vi "2013_02_13 Durability8 Main.vi"() -> ()   [LabVIEW 2012]
uses:
  MotorTypeDef.ctl
  <vilib>/DAQmx/write.llb/DAQmx Write (Counter Time 1Chan 1Samp).vi
  <vilib>/DAQmx/read.llb/DAQmx Read (Analog 1D Wfm NChan NSamp).vi
  <vilib>/Utility/TradDaqScaling.llb/Convert Thermistor Reading (waveform).vi
  <vilib>/DAQmx/miscellaneous.llb/DAQmx Fill In Error Info.vi
  <resource>/objmgr/daqmx.rc
panel:
  out "TotalSampPerChanAcquired":dbl
  out "AvailSampPerChan":u32
  in  "Y axis":u16(ring)=3 items=["RMS Current (A) 1"=1, "RMS Voltage (V) 1"=2, "RPM"=3, "Supply (V)"=4, "Torque (mNm)"=5, "Electrical Power (W)"=6, "Mechanical Power(W)"=7, "Motor Efficiency (%)"=8, "Source Current (A)"=10, "Supply Power (W)"=11, "ESC Efficiency (%)"=12, "Flow"=13, "Pressure Blue"=14, "Pressure Yellow"=15, "etc"=16]
  in  "X axis":u16(ring) items=["RMS Current (A) 1"=1, "RMS Voltage (V) 1"=2, "RPM"=3, "Supply (V)"=4, "Torque (mNm)"=5, "Electrical Power (W)"=6, "Mechanical Power(W)"=7, "Motor Efficiency (%)"=8, "Source Current (A)"=10, "Supply Power (W)"=11, "ESC Efficiency (%)"=12, "Flow"=13, "Pressure Blue"=14, "Pressure Yellow"=15, "Elapsed Time (s)"=0]
  out "XY Graph 2":cluster{"Array":dbl[], "Array":dbl[]}[](graph)
  out "Single Motor 2":waveform(dbl)[](graph)
  in  "Waveform":bool
  in  "Motor":dbl=1.0 min=1.0 max=8.0 step=1.0
  out "XY Graph":cluster{"Array":dbl[], "Array":dbl[]}[](graph)
  out "error out":errorcluster
  in  "File Path":path=path "Durability/.lvm"
  in  "Motor 8":T1 {"Elec Power In (W)" format="%.3g"; "Efficiency" format="%#_3g%%"; "Mech Pwr Out (W)" format="%.3g"; "Torque (mNm)" format="%.3g"; "Elapsed Time" format="%<%H:%M:%S>t"; "Supply (V)" format="%.2f"; "RPM" scale=0.0..40000.0 scale format="%#_4p"}
  in  "Motor 7":T1 {"Elec Power In (W)" format="%.3g"; "Efficiency" format="%#_3g%%"; "Mech Pwr Out (W)" format="%.3g"; "Torque (mNm)" format="%.3g"; "Elapsed Time" format="%<%H:%M:%S>t"; "Supply (V)" format="%.2f"; "RPM" scale=0.0..40000.0 scale format="%#_4p"}
  in  "Motor 6":T1 {"Elec Power In (W)" format="%.3g"; "Efficiency" format="%#_3g%%"; "Mech Pwr Out (W)" format="%.3g"; "Torque (mNm)" format="%.3g"; "Elapsed Time" format="%<%H:%M:%S>t"; "Supply (V)" format="%.2f"; "RPM" scale=0.0..40000.0 scale format="%#_4p"}
  in  "Motor 5":T1 {"Elec Power In (W)" format="%.3g"; "Efficiency" format="%#_3g%%"; "Mech Pwr Out (W)" format="%.3g"; "Torque (mNm)" format="%.3g"; "Elapsed Time" format="%<%H:%M:%S>t"; "Supply (V)" format="%.2f"; "RPM" scale=0.0..40000.0 scale format="%#_4p"}
  in  "Motor 4":T1 {"Elec Power In (W)" format="%.3g"; "Efficiency" format="%#_3g%%"; "Mech Pwr Out (W)" format="%.3g"; "Torque (mNm)" format="%.3g"; "Elapsed Time" format="%<%H:%M:%S>t"; "Supply (V)" format="%.2f"; "RPM" scale=0.0..40000.0 scale format="%#_4p"}
  in  "Motor 3":T1 {"Elec Power In (W)" format="%.3g"; "Efficiency" format="%#_3g%%"; "Mech Pwr Out (W)" format="%.3g"; "Torque (mNm)" format="%.3g"; "Elapsed Time" format="%<%H:%M:%S>t"; "Supply (V)" format="%.2f"; "RPM" scale=0.0..40000.0 scale format="%#_4p"}
  in  "Motor 2":T1 {"Elec Power In (W)" format="%.3g"; "Efficiency" format="%#_3g%%"; "Mech Pwr Out (W)" format="%.3g"; "Torque (mNm)" format="%.3g"; "Elapsed Time" format="%<%H:%M:%S>t"; "Supply (V)" format="%.2f"; "RPM" scale=0.0..40000.0 scale format="%#_4p"}
  in  "Motor 1":T1 {"Elec Power In (W)" format="%.3g"; "Efficiency" format="%#_3g%%"; "Mech Pwr Out (W)" format="%.3g"; "Torque (mNm)" format="%.3g"; "Elapsed Time" format="%<%H:%M:%S>t"; "Supply (V)" format="%.2f"; "RPM" scale=0.0..40000.0 scale format="%#_4p"}
  out "Motor Temp":dbl(slide) scale=65.0..110.0
  out "Tank Temp":dbl(slide) scale=65.0..110.0
  in  "Temp Probe\nOn Motor":dbl=9.0
  out "loop time (ms)":u32
  in  "stop":bool
  in  "Unlock PWM":bool=TRUE
  in  "PWM 2":dbl(slide)=100.0 min=0.0 max=100.0 step=5.0 scale=0.0..100.0
  in  "PWM 1":dbl(slide) min=0.0 max=100.0 step=5.0 scale=0.0..100.0
  # "Enable"
  # "Fail"
  # "Enable"
  # "Fail"
  # "Enable"
  # "Fail"
  # "Enable"
  # "Fail"
  # "Enable"
  # "Fail"
  # "Enable"
  # "Fail"
  # "Enable"
  # "Fail"
  # "Enable"
  # "Fail"
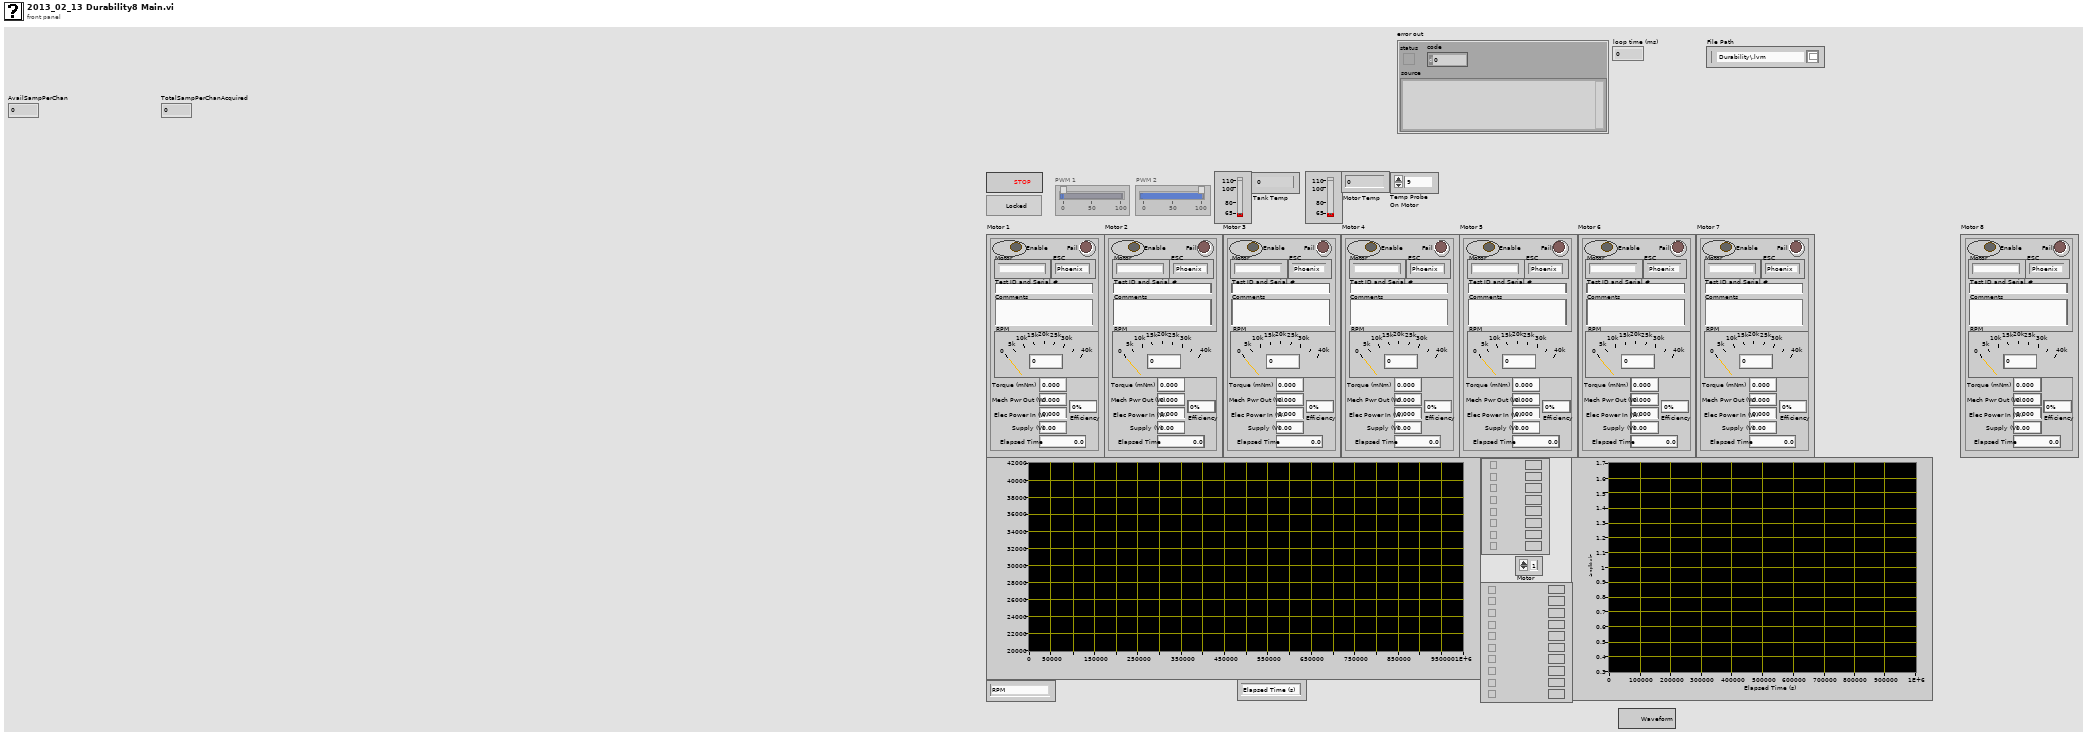
[diagram p1: front panel]
types:
  T1 = typedef "MotorTypeDef.ctl" = cluster{"Enabled":bool, "Fail":bool, "RPM":dbl, "Motor":enum16{"", "Maxon EC6 6V", "Maxon EC4 6V", "FH 0620 6V", "FH 0620 12V"}, "ESC":enum16{"Phoenix", "Maxon", "FH 1801"}, "Supply (V)":dbl, "Test ID and Serial #":string, "Comments":string, "Elapsed Time":dbl, "Counter":dbl, "Torque (mNm)":dbl, "Mech Pwr Out (W)":dbl, "Efficiency":dbl, "Elec Power In (W)":dbl}
  T2 = enum8{"Enabled", "Disabled", "Disabled and Grayed Out"}
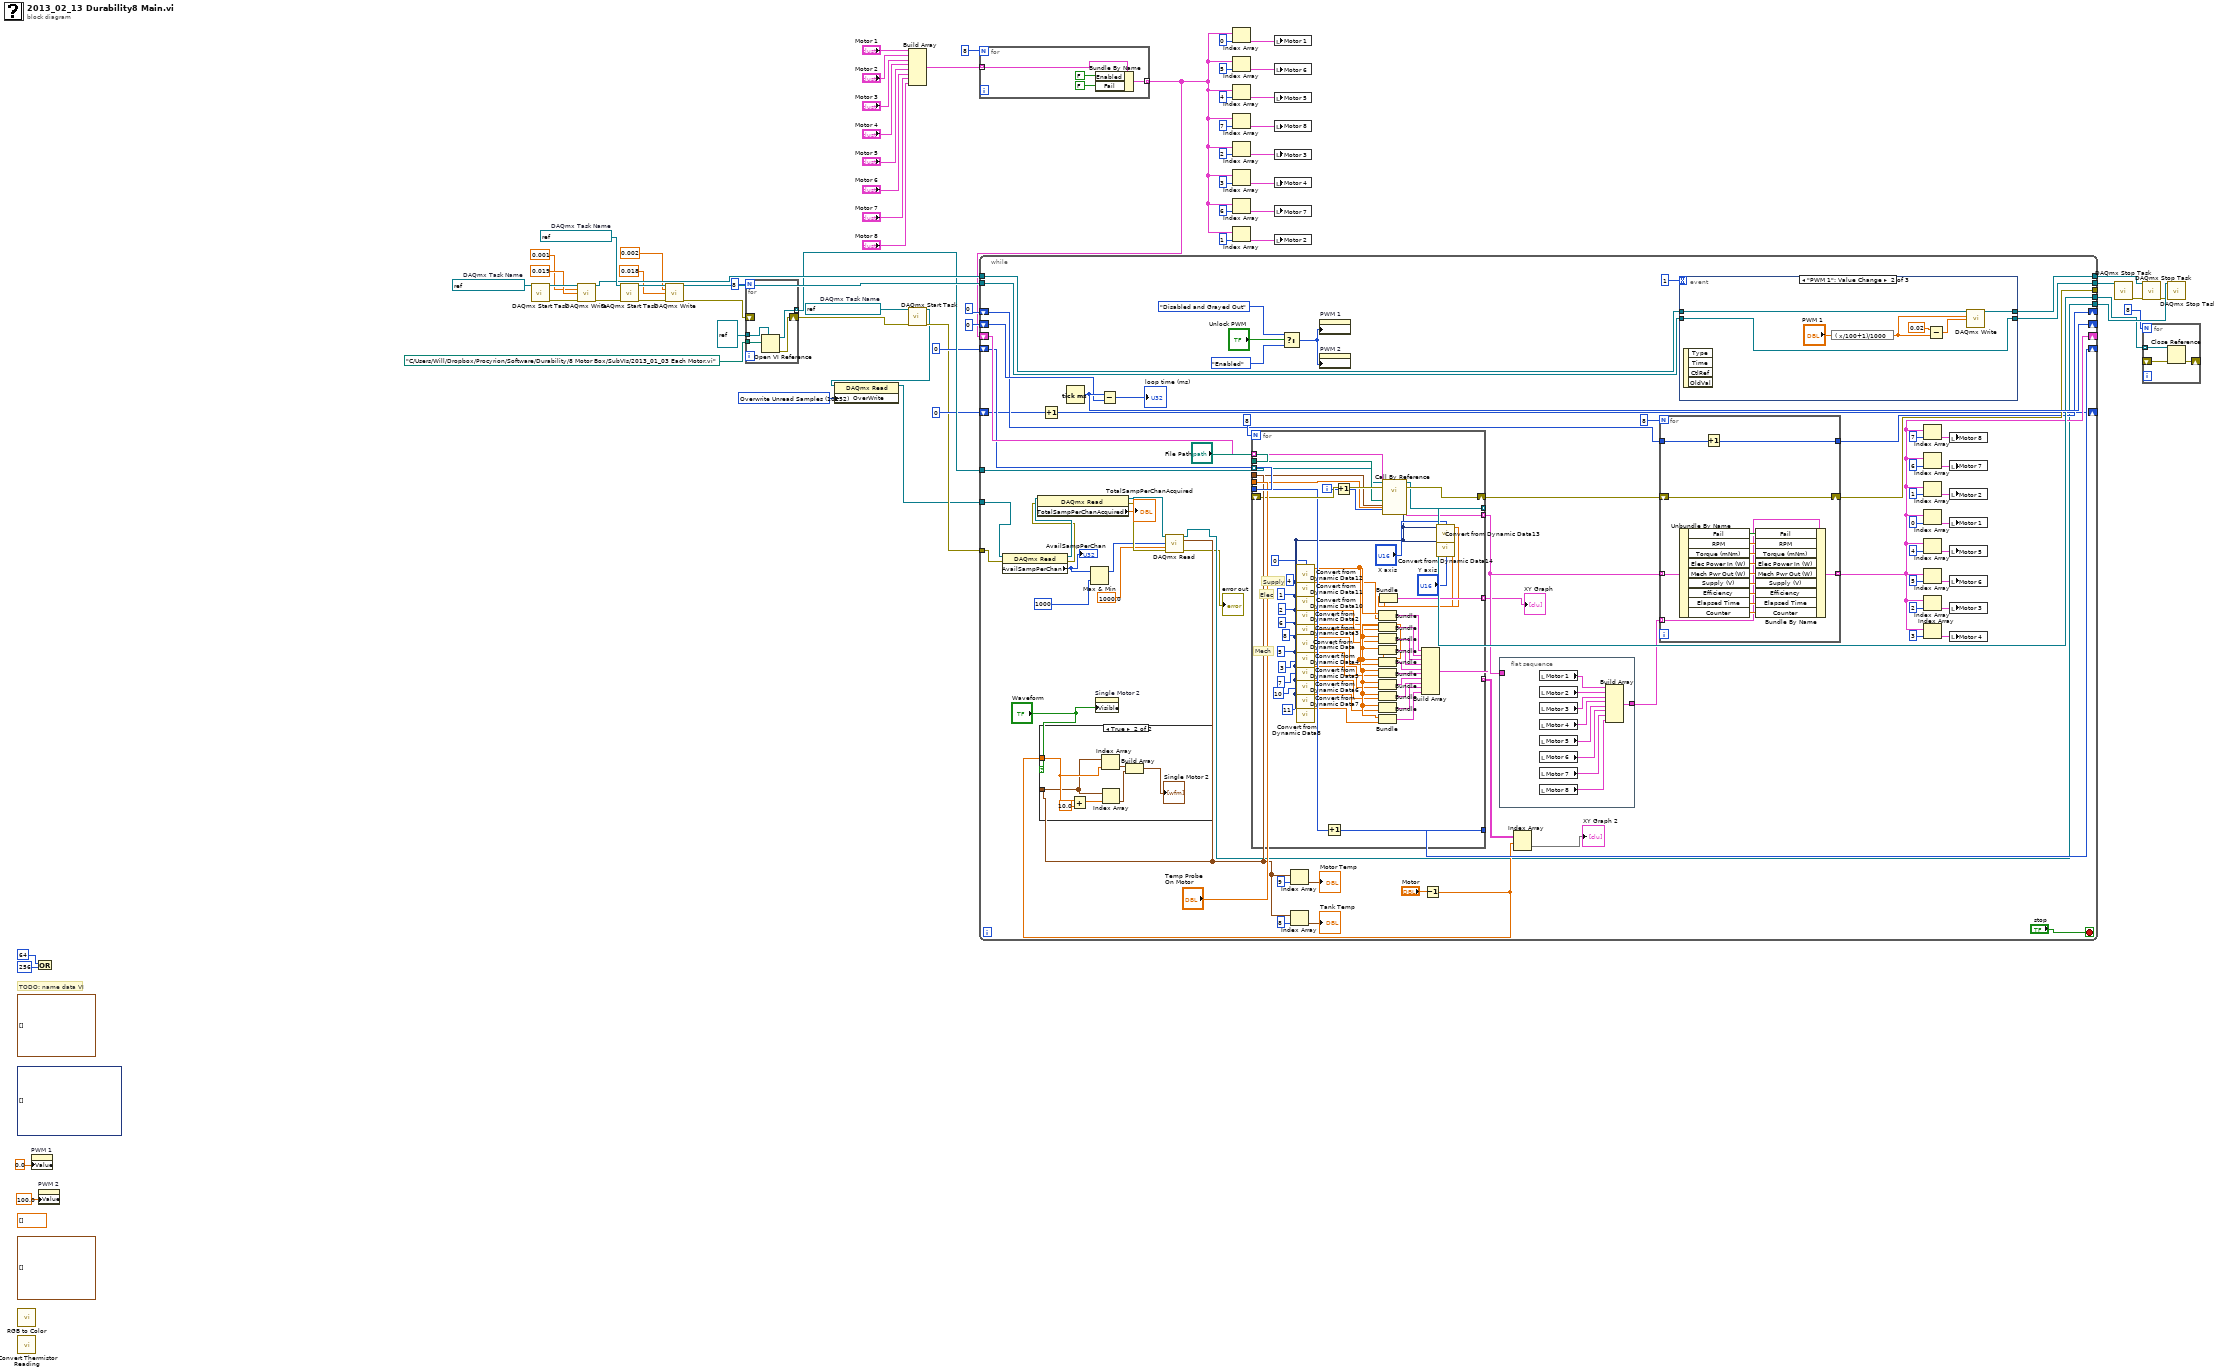
[diagram p0: block diagram]
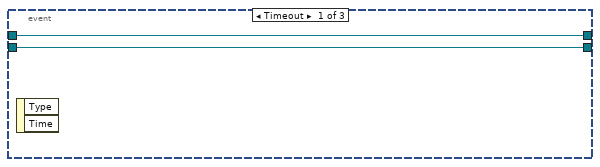
[diagram p3: hidden frame]
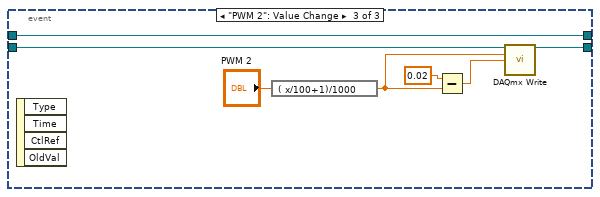
[diagram p4: hidden frame]
diagram:
  w1 = 10252 items=["Overwrite Unread Samples"=10252, "Do Not Overwrite Unread Samples"=10159] ("OverWrite")
  (unwired) dynamicdata[] []
  (unwired) dbl[] [] ("History Data")
  (unwired) waveform(dbl)[][] [] ("History Data")
  (unwired) waveform(dbl)[][] [] ("History Data")
  w63 = refnum<k21> "Durability8 PWM2"  # DAQmx Task Name
  w64 = refnum<k21> "Durability8 PWM1"  # DAQmx Task Name
  w66 = refnum<k21> "Durability8 Acquire"  # DAQmx Task Name
  # "TODO: name data VI"
  n1 = call <vilib>:"RGB to Color.vi"() -> ()  [unwired: 3 in, 1 out]
  n2 = call-poly <vilib>:"Convert Thermistor Reading.vi"() -> ()  [unwired: 7 in, 1 out]
  n3 = property on="PWM 1" class="Slide (strict)"("Value"=0.0 ("PWM 1")) -> ()  [unwired: 2 in, 2 out]
  n4 = Compound Arithmetic op=OR(64 ("options"), 256 ("options")) -> ()  [unwired: 1 out]
  n5 = property on="PWM 2" class="Slide (strict)"("Value"=100.0 ("PWM 2")) -> ()  [unwired: 2 in, 2 out]
  n6 = call <vilib>:"DAQmx Start Task.vi"("task/channels in"=w64) -> ("task out"=w60:refnum<k21>, "error out"=w58:errorcluster)  [unwired: 13 in]
  n7 = call-poly <vilib>:"DAQmx Write.vi"("task/channels in"=w60, "high time"=0.001 ("data"), "low time"=0.019 ("data"), "error in"=w58) -> ("task out"=w62:refnum<k21>, "error out"=w57:errorcluster)  [unwired: 9 in, 1 out]
  n8 = call <vilib>:"DAQmx Start Task.vi"("task/channels in"=w63, "error in"=w57) -> ("task out"=w59:refnum<k21>, "error out"=w56:errorcluster)  [unwired: 12 in]
  n9 = call-poly <vilib>:"DAQmx Write.vi"("task/channels in"=w59, "high time"=0.002 ("data"), "low time"=0.018 ("data"), "error in"=w56) -> ("task out"=w61:refnum<k21>, "error out"=w25:errorcluster)  [unwired: 9 in, 1 out]
  n10 = for {
    N: 8 -> [_]
    tunnel: path "C:/Users/Will/Dropbox/Procyrion/Software/Durability/8 Motor Box/SubVIs/2013_01_03 Each Motor.vi" -> [w70]
    tunnel: [w69] -> w41 mode=indexing
    tunnel: refnum<vi> refnum ("type specifier VI Refnum (for type only)") -> [w68]
    shift-right: [w67] -> w26
    shift-left: w25 -> [_]
    n11 = Open VI Reference(type specifier VI Refnum (for type only)=w68, vi path=w70) -> (vi reference=w69:refnum<vi>, error out=w67:errorcluster)  [unwired: 4 in]
  }
  n12 = Build Array("Motor 1", "Motor 2", "Motor 3", "Motor 4", "Motor 5", "Motor 6", "Motor 7", "Motor 8") -> (w22:T1[])
  n13 = call <vilib>:"DAQmx Start Task.vi"("task/channels in"=w66, "error in"=w26) -> ("task out"=w3:refnum<k21>, "error out"=w24:errorcluster)  [unwired: 12 in]
  n14 = property class="DAQmx Read"(reference=w3, "OverWrite"=w1) -> (reference out=w2:refnum<k21>)  [unwired: 1 in, 1 out]
  n15 = for {
    N: 8 -> [_]
    tunnel: w22 -> [w74] mode=indexing
    tunnel: [w71] -> w5 mode=indexing
    n16 = Bundle By Name(cluster=w74, "Enabled"=FALSE, "Fail"=FALSE) -> (w71:T1)
  }
  n17 = while {
    tunnel: w2 -> [w85]
    tunnel: [w89] -> w65
    tunnel: w24 -> [w84]
    shift-right: [w141] -> _
    shift-left: u32 0 ("millisecond timer value") -> [w140]
    tunnel: w62 -> [w133]
    tunnel: w61 -> [w132]
    tunnel: [w131] -> w55
    tunnel: [w130] -> w48
    tunnel: w41 -> [w126]
    tunnel: [w125] -> w37
    shift-right: [w107] -> _
    shift-left: w5 -> [w106]
    tunnel: [w105] -> _
    shift-right: [w102] -> _
    shift-left: 0 ("for") -> [w103]
    shift-right: [w100] -> _
    shift-left: 0 ("for") -> [w101]
    shift-right: [w98] -> _
    shift-left: 0 ("for") -> [w99]
    stop <- "stop" stop-if-true
    n18 = property class="DAQmx Read"(reference=w85, error in=w84) -> (reference out=w83:refnum<k21>, error out=w82:errorcluster, "AvailSampPerChan"=w81:u32)
    "AvailSampPerChan" <- w81
    n19 = property class="DAQmx Read"(reference=w83, error in=w82) -> (reference out=w79:refnum<k21>, error out=w78:errorcluster, "TotalSampPerChanAcquired"=→"TotalSampPerChanAcquired":dbl)
    n20 = Increment(x=w99) -> (x+1=w98:i32)
    n21 = Tick Count (ms)() -> (millisecond timer value=w141:u32)
    n22 = Max & Min(x=w81, y=1000 ("number of samples per channel")) -> (max(x,y)=w76:u32)  [unwired: 1 out]
    n23 = property on="Single Motor 2" class="WFGraph (strict)"("Visible"="Waveform") -> ()  [unwired: 2 in, 2 out]
    n24 = Subtract(x=w141, y=w140) -> (x-y=→"loop time (ms)":u32)
    n25 = call-poly <vilib>:"DAQmx Read.vi"("task/channels in"=w79, "number of samples per channel"=w76, "timeout"=1000.0, "error in"=w78) -> ("task out"=w89:refnum<k21>, "data"=w92:waveform(dbl)[], "error out"=→"error out":errorcluster)  [unwired: 9 in]
    n26 = for {
      N: 8 -> [_]
      tunnel: w92 -> [w240]
      tunnel: "File Path" -> [w241]
      tunnel: w126 -> [w205] mode=indexing
      shift-right: [w244] -> w104
      shift-left: _ -> [w243]
      tunnel: [w238] -> w125 mode=indexing
      tunnel: [w237] -> w96 mode=indexing
      tunnel: w106 -> [w193] mode=indexing
      tunnel: w103 -> [w236]
      tunnel: [w235] -> w102
      tunnel: "Temp Probe\nOn Motor" -> [w234]
      tunnel: [w233] -> w94 mode=indexing
      tunnel: [w221] -> w88 mode=indexing
      i -> [w242]
      # "Mech"
      # "Elec"
      # "Supply"
      n27 = Increment(x=w236) -> (x+1=w235:i32)
      n28 = Increment(x=w242) -> (x+1=w239:i32)
      n29 = call-by-ref "?"(reference=w205, error in=w243, "Temp On"=w234, "Motor #"=w239, "data"=w240, "File Path"=w241, "Motor Typedef"=w193) -> (reference out=w238:refnum<vi>, error out=w244:errorcluster, "Final Out"=w208:dynamicdata, "Motor Typedef Out"=w237:T1)  [unwired: 5 in]
      n30 = call "Convert from Dynamic Data12"("Dynamic Data Type"=w208, "Channel"=0) -> ("Array"=w222:dbl[])  [unwired: 2 in]
      n31 = call "Convert from Dynamic Data11"("Dynamic Data Type"=w208, "Channel"=4) -> ("Array"=w220:dbl[])  [unwired: 2 in]
      n32 = call "Convert from Dynamic Data10"("Dynamic Data Type"=w208, "Channel"=1) -> ("Array"=w219:dbl[])  [unwired: 2 in]
      n33 = call "Convert from Dynamic Data2"("Dynamic Data Type"=w208, "Channel"=2) -> ("Array"=w218:dbl[])  [unwired: 2 in]
      n34 = call "Convert from Dynamic Data3"("Dynamic Data Type"=w208, "Channel"=6) -> ("Array"=w217:dbl[])  [unwired: 2 in]
      n35 = call "Convert from Dynamic Data"("Dynamic Data Type"=w208, "Channel"=8) -> ("Array"=w216:dbl[])  [unwired: 2 in]
      n36 = call "Convert from Dynamic Data4"("Dynamic Data Type"=w208, "Channel"=5) -> ("Array"=w215:dbl[])  [unwired: 2 in]
      n37 = call "Convert from Dynamic Data5"("Dynamic Data Type"=w208, "Channel"=3) -> ("Array"=w214:dbl[])  [unwired: 2 in]
      n38 = call "Convert from Dynamic Data6"("Dynamic Data Type"=w208, "Channel"=7) -> ("Array"=w213:dbl[])  [unwired: 2 in]
      n39 = call "Convert from Dynamic Data7"("Dynamic Data Type"=w208, "Channel"=10) -> ("Array"=w212:dbl[])  [unwired: 2 in]
      n40 = call "Convert from Dynamic Data8"("Dynamic Data Type"=w208, "Channel"=11) -> ("Array"=w211:dbl[])  [unwired: 2 in]
      n41 = Bundle("Array"=w222, "Array"=w220) -> (w223:cluster{"Array":dbl[], "Array":dbl[]})  [unwired: 1 in]
      n42 = Bundle("Array"=w222, "Array"=w219) -> (w224:cluster{"Array":dbl[], "Array":dbl[]})  [unwired: 1 in]
      n43 = Bundle("Array"=w222, "Array"=w218) -> (w225:cluster{"Array":dbl[], "Array":dbl[]})  [unwired: 1 in]
      n44 = Bundle("Array"=w222, "Array"=w217) -> (w226:cluster{"Array":dbl[], "Array":dbl[]})  [unwired: 1 in]
      n45 = Bundle("Array"=w222, "Array"=w216) -> (w227:cluster{"Array":dbl[], "Array":dbl[]})  [unwired: 1 in]
      n46 = Bundle("Array"=w222, "Array"=w215) -> (w228:cluster{"Array":dbl[], "Array":dbl[]})  [unwired: 1 in]
      n47 = Bundle("Array"=w222, "Array"=w214) -> (w229:cluster{"Array":dbl[], "Array":dbl[]})  [unwired: 1 in]
      n48 = Bundle("Array"=w222, "Array"=w213) -> (w230:cluster{"Array":dbl[], "Array":dbl[]})  [unwired: 1 in]
      n49 = Bundle("Array"=w222, "Array"=w212) -> (w232:cluster{"Array":dbl[], "Array":dbl[]})  [unwired: 1 in]
      n50 = Bundle("Array"=w222, "Array"=w211) -> (w231:cluster{"Array":dbl[], "Array":dbl[]})  [unwired: 1 in]
      n51 = Build Array(w223, w224, w225, w226, w227, w228, w229, w230, w232, w231) -> (w221:cluster{"Array":dbl[], "Array":dbl[]}[])
      n52 = call "Convert from Dynamic Data13"("Dynamic Data Type"=w208, "Channel"="X axis") -> ("Array"=w207:dbl[])  [unwired: 2 in]
      n53 = call "Convert from Dynamic Data14"("Dynamic Data Type"=w208, "Channel"="Y axis") -> ("Array"=w206:dbl[])  [unwired: 2 in]
      n54 = Bundle("Array"=w207, "Array"=w206) -> (w233:cluster{"Array":dbl[], "Array":dbl[]})  [unwired: 1 in]
    }
    "XY Graph" <- w94
    n55 = Select(t=T2."Disabled and Grayed Out" ("Disabled"), s="Unlock PWM", f=T2."Enabled" ("Disabled")) -> (s? t:f=w145:T2)
    n56 = Index Array(array=w92, index=9) -> (element=→"Motor Temp":waveform(dbl))
    n57 = Index Array(array=w92, index=8) -> (element=→"Tank Temp":waveform(dbl))
    n58 = property on="PWM 1" class="Slide (strict)"("DisabledEnum"=w145) -> ()  [unwired: 2 in, 2 out]
    n59 = property on="PWM 2" class="Slide (strict)"("DisabledEnum"=w145) -> ()  [unwired: 2 in, 2 out]
    n60 = Decrement(x="Motor") -> (x-1=w91:dbl)
    n61 = case shown="True" "Waveform" {
      tunnel: w92 -> [_ w150]
      tunnel: w91 -> [_ w151]
      frame False {
      }
      frame True {
        n62 = Add(x=w151, y=10.0) -> (x+y=w149:dbl)
        n63 = Index Array(array=w150, index=w151) -> (element=w148:waveform(dbl))
        n64 = Index Array(array=w150, index=w149) -> (element=w147:waveform(dbl))
        n65 = Build Array(w148, w147) -> (→"Single Motor 2":waveform(dbl)[])
      }
    }
    n66 = flat-sequence {
      tunnel: [w154] -> w97
      tunnel: w96 -> [_]
      frame #0 {
        n67 = local read "Motor 1"() -> (w155:T1)
        n68 = local read "Motor 2"() -> (w156:T1)
        n69 = local read "Motor 3"() -> (w157:T1)
        n70 = local read "Motor 4"() -> (w158:T1)
        n71 = local read "Motor 5"() -> (w159:T1)
        n72 = local read "Motor 6"() -> (w160:T1)
        n73 = local read "Motor 7"() -> (w161:T1)
        n74 = local read "Motor 8"() -> (w153:T1)
        n75 = Build Array(w155, w156, w157, w158, w159, w160, w161, w153) -> (w154:T1[])
      }
    }
    n76 = Index Array(array=w88, index (row)=w91) -> (element=→"XY Graph 2":cluster{"Array":dbl[], "Array":dbl[]}[])  [unwired: 1 in]
    n77 = for {
      N: 8 -> [_]
      tunnel: w97 -> [w167] mode=indexing
      tunnel: [w166] -> w107 mode=indexing
      tunnel: w96 -> [w165] mode=indexing
      shift-right: [w164] -> w105
      shift-left: w104 -> [w164]
      tunnel: [w162] -> w100
      tunnel: w101 -> [w163]
      n78 = Unbundle By Name(w165) -> ("Fail"=w176:bool, "RPM"=w175:dbl, "Torque (mNm)"=w174:dbl, "Elec Power In (W)"=w173:dbl, "Mech Pwr Out (W)"=w172:dbl, "Supply (V)"=w171:dbl, "Efficiency"=w170:dbl, "Elapsed Time"=w169:dbl, "Counter"=w168:dbl)
      n79 = Increment(x=w163) -> (x+1=w162:i32)
      n80 = Bundle By Name(cluster=w167, "Fail"=w176, "RPM"=w175, "Torque (mNm)"=w174, "Elec Power In (W)"=w173, "Mech Pwr Out (W)"=w172, "Supply (V)"=w171, "Efficiency"=w170, "Elapsed Time"=w169, "Counter"=w168) -> (w166:T1)
    }
    n81 = event shown="[1] \"PWM 1\": Value Change" {
      selector: _ -> [_ _ _]
      dyn-events: _ -> [_ _ _]
      timeout: 1 -> [_ _ _]
      tunnel: w133 -> [w178 w181 w187]
      tunnel: w132 -> [w177 w179 w186]
      tunnel: [w178 w180 w187] -> w131
      tunnel: [w177 w179 w188] -> w130
      event Timeout {
        n82 = event-data() -> ()  [unwired: 1 in, 2 out]
      }
      event "PWM 1": Value Change {
        n83 = event-data() -> ()  [unwired: 1 in, 4 out]
        n84 = expression code="( x/100+1)/1000"("PWM 1") -> (w182:dbl)
        n85 = Subtract(x=0.02 ("y"), y=w182) -> (x-y=w183:dbl)
        n86 = call-poly <vilib>:"DAQmx Write.vi"("task/channels in"=w181, "high time"=w182, "low time"=w183) -> ("task out"=w180:refnum<k21>)  [unwired: 10 in, 2 out]
      }
      event "PWM 2": Value Change {
        n87 = event-data() -> ()  [unwired: 1 in, 4 out]
        n88 = expression code="( x/100+1)/1000"("PWM 2") -> (w192:dbl)
        n89 = Subtract(x=0.02, y=w192) -> (x-y=w190:dbl)
        n90 = call-poly <vilib>:"DAQmx Write.vi"("task/channels in"=w186, "high time"=w192, "low time"=w190) -> ("task out"=w188:refnum<k21>)  [unwired: 10 in, 2 out]
      }
    }
    n91 = Index Array(array=w107, index=7) -> (element=w114:T1)
    n92 = Index Array(array=w107, index=6) -> (element=w113:T1)
    n93 = Index Array(array=w107, index=1) -> (element=w108:T1)
    n94 = Index Array(array=w107, index=0) -> (element=w123:T1)
    n95 = Index Array(array=w107, index=4) -> (element=w111:T1)
    n96 = Index Array(array=w107, index=5) -> (element=w112:T1)
    n97 = Index Array(array=w107, index=2) -> (element=w109:T1)
    n98 = Index Array(array=w107, index=3) -> (element=w110:T1)
    n99 = local write "Motor 8"(w114) -> ()
    n100 = local write "Motor 7"(w113) -> ()
    n101 = local write "Motor 2"(w108) -> ()
    n102 = local write "Motor 1"(w123) -> ()
    n103 = local write "Motor 5"(w111) -> ()
    n104 = local write "Motor 6"(w112) -> ()
    n105 = local write "Motor 3"(w109) -> ()
    n106 = local write "Motor 4"(w110) -> ()
  }
  n107 = Index Array(array=w5, index=0) -> (element=w21:T1)
  n108 = Index Array(array=w5, index=5) -> (element=w10:T1)
  n109 = Index Array(array=w5, index=4) -> (element=w9:T1)
  n110 = Index Array(array=w5, index=7) -> (element=w12:T1)
  n111 = Index Array(array=w5, index=2) -> (element=w7:T1)
  n112 = Index Array(array=w5, index=3) -> (element=w8:T1)
  n113 = Index Array(array=w5, index=6) -> (element=w11:T1)
  n114 = Index Array(array=w5, index=1) -> (element=w6:T1)
  n115 = local write "Motor 1"(w21) -> ()
  n116 = local write "Motor 6"(w10) -> ()
  n117 = local write "Motor 5"(w9) -> ()
  n118 = local write "Motor 8"(w12) -> ()
  n119 = local write "Motor 3"(w7) -> ()
  n120 = local write "Motor 4"(w8) -> ()
  n121 = local write "Motor 7"(w11) -> ()
  n122 = local write "Motor 2"(w6) -> ()
  n123 = call <vilib>:"DAQmx Stop Task.vi"("task/channels in"=w48) -> ("error out"=w54:errorcluster)  [unwired: 13 in, 1 out]
  n124 = call <vilib>:"DAQmx Stop Task.vi"("task/channels in"=w55, "error in"=w54) -> ("error out"=w53:errorcluster)  [unwired: 12 in, 1 out]
  n125 = for {
    N: 8 -> [_]
    shift-right: [w247] -> _
    shift-left: _ -> [w245]
    tunnel: w37 -> [w246] mode=indexing
    n126 = Close Reference(reference=w246, error in (no error)=w245) -> (error out=w247:errorcluster)
  }
  n127 = call <vilib>:"DAQmx Stop Task.vi"("task/channels in"=w65, "error in"=w53) -> ()  [unwired: 12 in, 2 out]
